vi "FIFO Check_2.vi"(0 "FPGA Ref in":T3, 5 "Read at least # points":u32, 7 "Imaging Protocol":T1, 9 "Target number of points":u64, 11 "error in (no error)":errorcluster, 12 "Force read":bool) -> (4 "FPGA Ref out":T3, 6 "Elements Available":T2, 8 "Both channels no more data (delayed by 1 iteration)":bool, 10 "Data available or data has just completed (read the FIFO)":bool, 15 "error out":errorcluster)   [LabVIEW 2020]
uses:
  RIG-SPECIFIC FILES/FPGA Refs/FPGA Ref.ctl
  Acquisition/Typedefs/FIFO elements available.ctl
  Typedefs/Imaging Protocols enum.ctl
  <vilib>/Utility/error.llb/Error Cluster From Error Code.vi
  <vilib>/rvi/errors/niLvFpgaAdjustHostInterfaceError.vi
  <vilib>/rvi/interface/nirviMethod/nirviMethod.xnode
  <vilib>/rvi/errors/niLvFpgaMergeErrorWithErrorCode.vi
  <vilib>/FPGAPlugInAG/Dynamic/niLvFpga_ReadFifo_Dynamic.vi
panel:
  out "No more data Ch1":bool
  out "No more data Ch0":bool
  out "Registered peak value":dbl
  in  "Timeout (ms)":i32=30
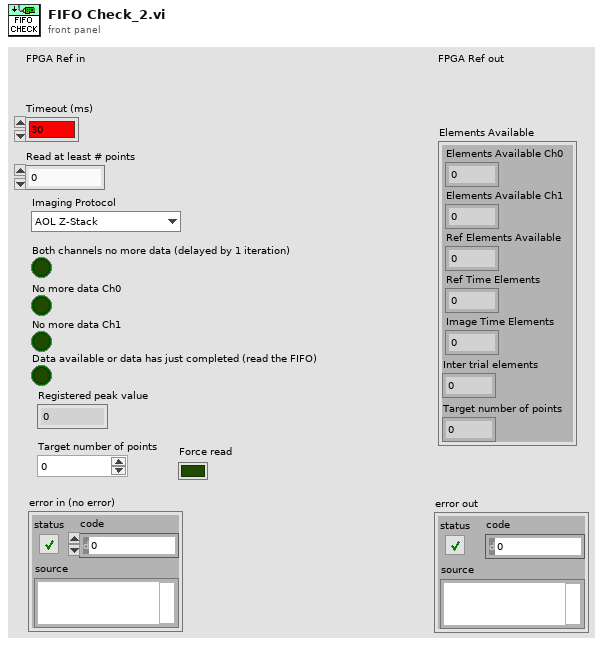
[diagram p1: front panel]
types:
  T1 = typedef "Imaging Protocols enum.ctl" = enum16{"AOL Z-Stack", "Motor Z Stack", "Functional Acquisition", "Single Plane Acquisition", "Volume Acquisition", "Live Imaging", "Live Plane Imaging", "Live Volume Imaging"}
  T2 = typedef "FIFO elements available.ctl" = cluster{"Elements Available Ch0":u32, "Elements Available Ch1":u32, "Ref Elements Available":u32, "Ref Time Elements":u32, "Image Time Elements":u32, "Inter trial elements":u32, "Target number of points":u64}
  T3 = typedef "FPGA Ref.ctl" = refnum<k20>
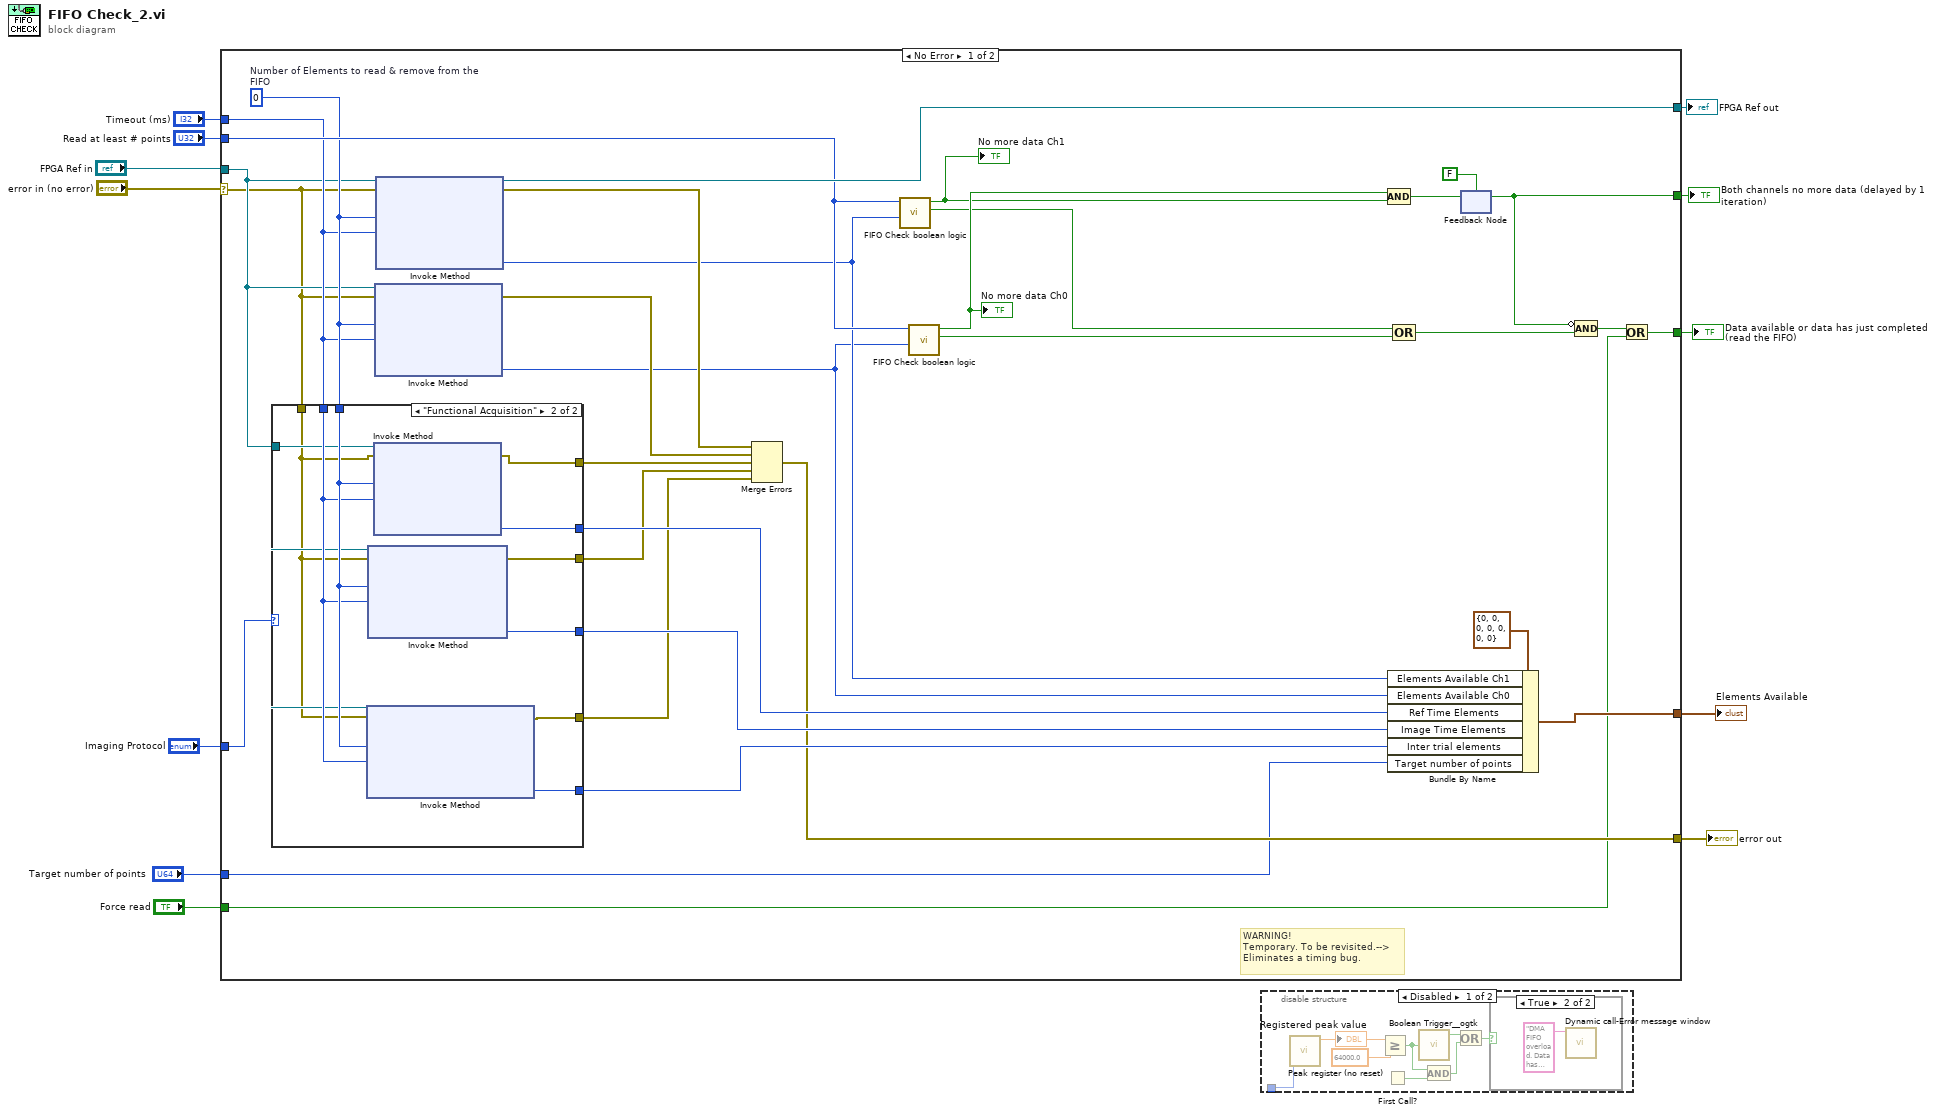
[diagram p0: block diagram]
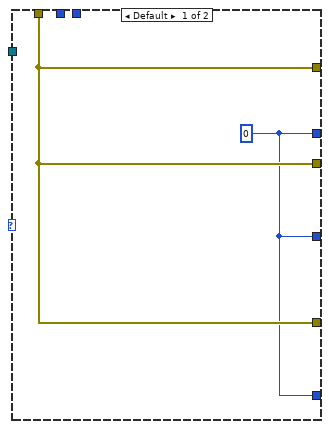
[diagram p2: hidden frame]
diagram:
  n1 = case shown="No Error" "error in (no error)" {
    selector: "error in (no error)" -> [w26 w58]
    tunnel: [w15 _] -> w12
    tunnel: [w44 w57] -> w11
    tunnel: "FPGA Ref in" -> [w27 w57]
    tunnel: "Timeout (ms)" -> [w30 _]
    tunnel: [w20 w58] -> w8
    tunnel: "Read at least # points" -> [w43 _]
    tunnel: [w42 _] -> w4
    tunnel: [w35 _] -> w5
    tunnel: "Imaging Protocol" -> [w18 _]
    tunnel: "Target number of points" -> [w17 _]
    tunnel: "Force read" -> [w13 _]
    frame No Error {
      w31 = u32 0  # Number of Elements to read & remove from the FIFO
      # "WARNING!\nTemporary. To be revisited.-->\nEliminates a timing bug."
      n2 = case shown="\"Functional Acquisition\"" w18 {
        tunnel: [w45 w56] -> w34
        tunnel: [w45 w55] -> w32
        tunnel: w31 -> [_ w54]
        tunnel: w30 -> [_ w53]
        tunnel: [w45 w52] -> w29
        tunnel: w27 -> [_ w51]
        tunnel: w26 -> [w46 w50]
        tunnel: [w46 w49] -> w23
        tunnel: [w46 w48] -> w22
        tunnel: [w46 w47] -> w21
        frame Default {
          w45 = u32 0 ("Elements Remaining")
        }
        frame "Functional Acquisition" {
          n3 = xnode ("Invoke Method")("FPGA VI Reference In"=w51, "error in"=w50, "Number of Elements"=w54, "Timeout (ms)"=w53) -> ("error out"=w47:errorcluster, "Elements Remaining"=w52:u32)  [unwired: 2 out]
          n4 = xnode ("Invoke Method")("FPGA VI Reference In"=w51, "error in"=w50, "Number of Elements"=w54, "Timeout (ms)"=w53) -> ("error out"=w48:errorcluster, "Elements Remaining"=w55:u32)  [unwired: 2 out]
          n5 = xnode ("Invoke Method")("FPGA VI Reference In"=w51, "error in"=w50, "Number of Elements"=w54, "Timeout (ms)"=w53) -> ("error out"=w49:errorcluster, "Elements Remaining"=w56:u32)  [unwired: 2 out]
        }
      }
      n6 = xnode ("Invoke Method")("FPGA VI Reference In"=w27, "error in"=w26, "Number of Elements"=w31, "Timeout (ms)"=w30) -> ("error out"=w24:errorcluster, "Elements Remaining"=w14:u32)  [unwired: 2 out]
      n7 = xnode ("Invoke Method")("FPGA VI Reference In"=w27, "error in"=w26, "Number of Elements"=w31, "Timeout (ms)"=w30) -> ("FPGA VI Reference Out"=w44:T3, "error out"=w25:errorcluster, "Elements Remaining"=w19:u32)  [unwired: 1 out]
      n8 = Merge Errors(w25, w24, w23, w22, w21) -> (w20:errorcluster)
      n9 = call "FIFO Check boolean logic.vi"("Elements Remaining"=w19, "Read at least"=w43) -> ("Read FIFO"=w28:bool, "No more data"=w39:bool)  [unwired: 8 in]
      "No more data Ch1" <- w39
      n10 = call "FIFO Check boolean logic.vi"("Elements Remaining"=w14, "Read at least"=w43) -> ("Read FIFO"=w41:bool, "No more data"=w40:bool)  [unwired: 8 in]
      "No more data Ch0" <- w40
      n11 = Compound Arithmetic op=AND(w40, w39) -> (w38:bool)
      n12 = Bundle By Name(cluster=T2 {"Elements Available Ch0"=0, "Elements Available Ch1"=0, "Ref Elements Available"=0, "Ref Time Elements"=0, "Image Time Elements"=0, "Inter trial elements"=0, "Target number of points"=0} ("Elements Available 2"), "Elements Available Ch1"=w19, "Elements Available Ch0"=w14, "Ref Time Elements"=w34, "Image Time Elements"=w32, "Inter trial elements"=w29, "Target number of points"=w17) -> (w42:T2)
      n13 = Compound Arithmetic op=OR(w28, w41) -> (w36:bool)
      n14 = feedback-in #1(w38) -> ()
      n15 = feedback #1(FALSE) -> (w35:bool)
      n16 = Compound Arithmetic op=AND(invert w35, w36) -> (w16:bool)
      n17 = Or(x=w16, y=w13) -> (x .or. y?=w15:bool)
    }
    frame Error {
    }
  }
  "error out" <- w8
  "FPGA Ref out" <- w11
  "Data available or data has just completed (read the FIFO)" <- w12
  "Both channels no more data (delayed by 1 iteration)" <- w5
  "Elements Available" <- w4
  n18 = disable-structure "Diagram Disable Structure" shown="Disabled" {
    disable-tunnel: _ -> [w66 _]
    frame Disabled {
      n19 = call <userlib>:"Peak register (no reset).vi"("Value in"=w66) -> ("Registered peak value"=w65:dbl)  [unwired: 10 in]
      "Registered peak value" <- w65
      n20 = Greater Or Equal?(x=w65, y=64000.0) -> (x >= y?=w63:bool)
      n21 = First Call?() -> (First Call?: T/F=w62:bool)
      n22 = call <userlib>:"Boolean Trigger__ogtk.vi"("Boolean Input"=w63) -> ("Rising Edge"=w61:bool)  [unwired: 1 in, 1 out]
      n23 = And(x=w63, y=w62) -> (x .and. y?=w60:bool)
      n24 = Or(x=w61, y=w60) -> (x .or. y?=w59:bool)
      n25 = case shown="True" w59 {
        frame False {
        }
        frame True {
          n26 = call "Dynamic call-Error message window.vi"("Error Message"="DMA FIFO overload. Data has been lost.") -> ()  [unwired: 10 in, 1 out]
        }
      }
    }
    frame Enabled {
    }
  }
